vi "HFR500 Check comms.vi"(3 "Channel Name String":string) -> (1 "Comms Channel Number":i32)   [LabVIEW 2022 SP3]
uses:
  HFR500 ppm Range.ctl
  Globals/Meas_global.vi
panel:
  out "Testing Ch Number":i32
  out "Number of Black Box file reads":i32
  out "Channel  number with good response":i32[](array[numeric])
  out "Channel numbers being polled":i32
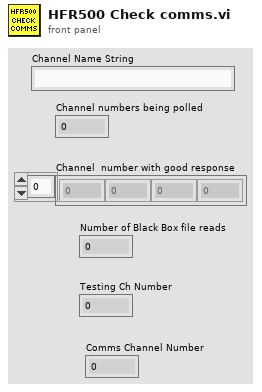
[diagram p1: front panel]
types:
  T1 = typedef "HFR500 ppm Range.ctl" = enum16{"None", "1,000", "2,000", "5,000", "10,000", "20,000", "50,000", "100,000", "200,000"}
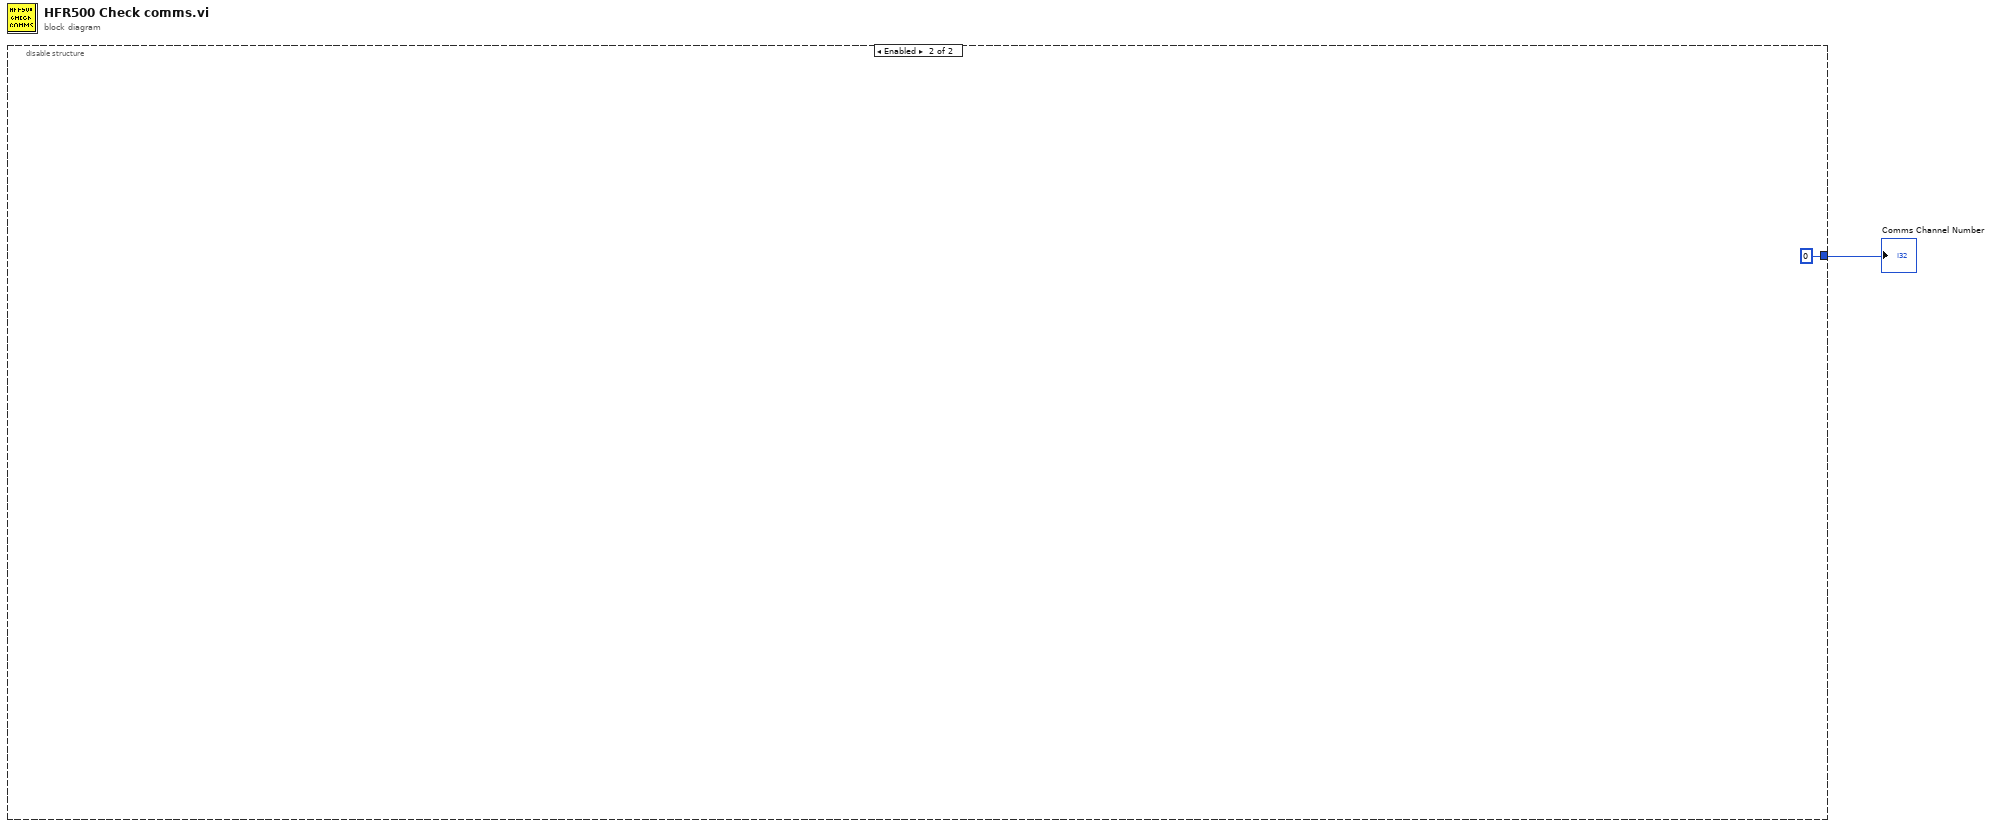
[diagram p0: block diagram]
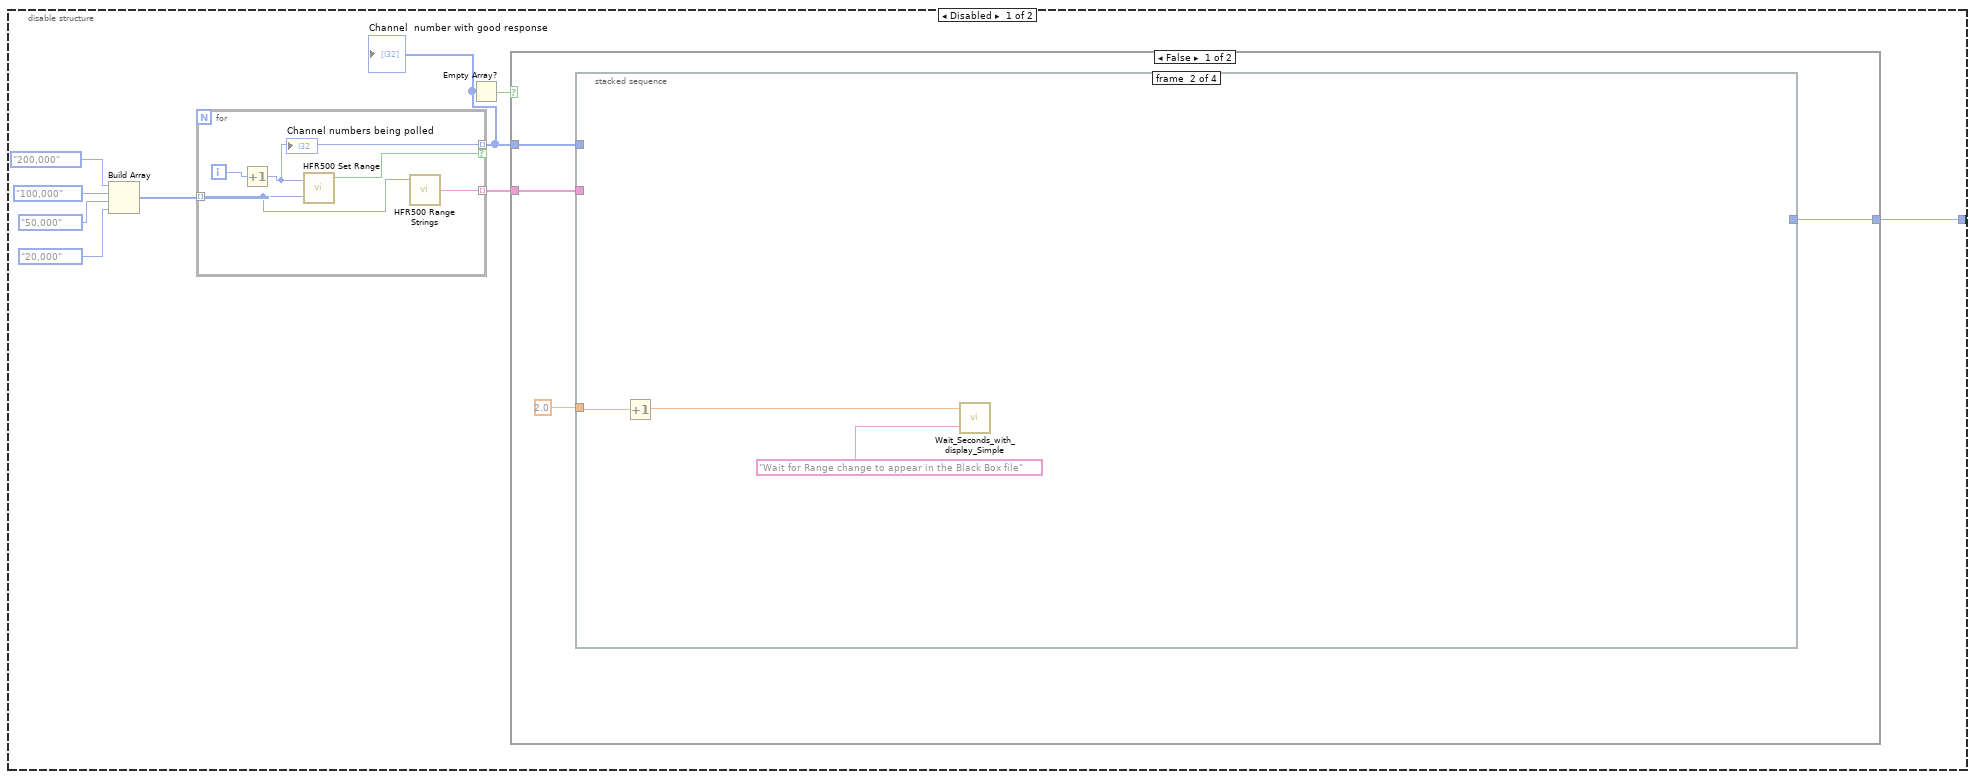
[diagram p2: hidden frame]
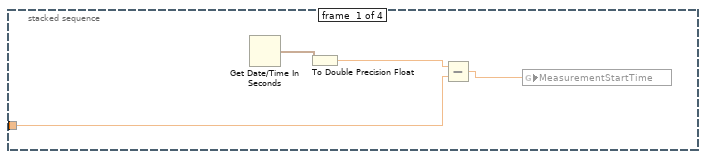
[diagram p3: hidden frame]
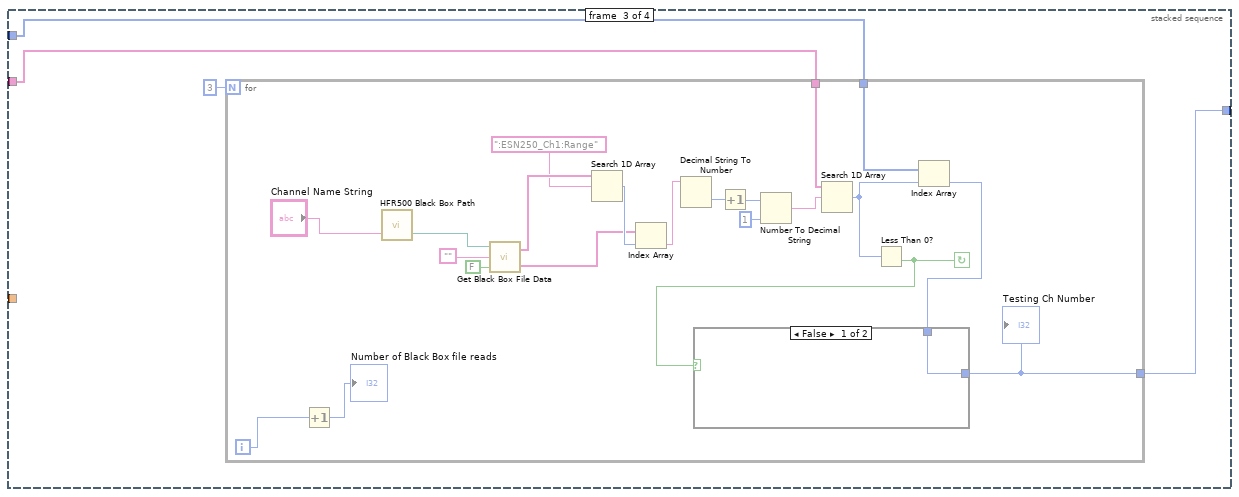
[diagram p4: hidden frame]
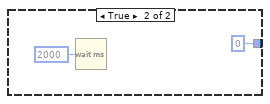
[diagram p5: hidden frame]
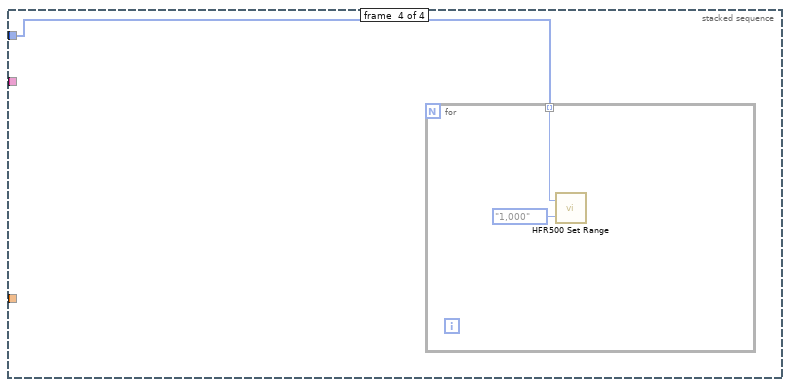
[diagram p6: hidden frame]
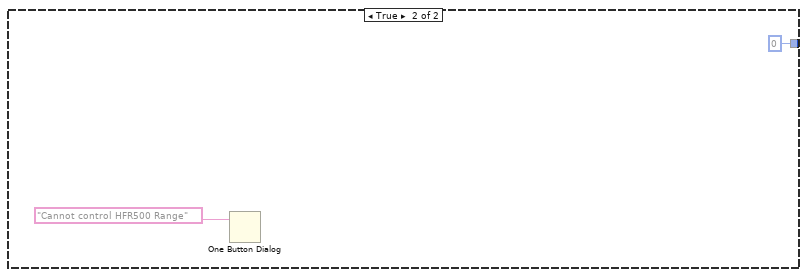
[diagram p7: hidden frame]
diagram:
  n1 = disable-structure shown="Enabled" {
    disable-tunnel: [w2 0 ("Comms Channel Number")] -> w1
    frame Disabled {
      n2 = Build Array(HFR500_ppm_Range."200,000" ("ppm Range"), HFR500_ppm_Range."100,000" ("ppm Range"), HFR500_ppm_Range."50,000" ("ppm Range"), HFR500_ppm_Range."20,000" ("ppm Range")) -> (w10:T1[])
      n3 = for {
        tunnel: w10 -> [w58] mode=indexing
        tunnel: [w57] -> w3 mode=indexing if=w56
        tunnel: [w55] -> w5 mode=indexing
        i -> [w59]
        n4 = Increment(x=w59) -> (x+1=w57:i32)
        "Channel numbers being polled" <- w57
        n5 = call "HFR500 Set Range.vi"("Ch number"=w57, "ppm Range"=w58) -> ("Correctly Set?"=w56:bool)  [unwired: 2 out]
        n6 = call "HFR500 Range Strings.vi"("ppm Range"=w58) -> ("Range Digit"=w55:string)  [unwired: 3 in, 1 out]
      }
      "Channel  number with good response" <- w3
      n7 = Empty Array?(array=w3) -> (empty?=w4:bool)
      n8 = case shown="False" w4 {
        tunnel: w3 -> [w13 _]
        tunnel: w5 -> [w12 _]
        tunnel: [w11 0] -> w2
        frame False {
          n9 = stacked-sequence {
            tunnel: 2.0 ("y") -> [w15 w21 _ _]
            tunnel: w13 -> [_ _ w24 w50]
            tunnel: w12 -> [_ _ w23 _]
            tunnel: [_ _ w22 _] -> w11
            frame #0 {
              n10 = Get Date/Time In Seconds() -> (seconds since 1Jan1904=w18:timestamp)
              n11 = To Double Precision Float(number=w18) -> (double precision float=w16:dbl)
              n12 = Subtract(x=w16, y=w15) -> (x-y=w17:dbl)
              n13 = global write "Meas_global.vi" "MeasurementStartTime"(w17) -> ()
            }
            frame #1 {
              n14 = Increment(x=w21) -> (x+1=w19:dbl)
              n15 = call "Wait_Seconds_with_display_Simple.vi"("Message"="Wait for Range change to appear in the Black Box file", "Seconds to wait"=w19) -> ()  [unwired: 1 in, 1 out]
            }
            frame #2 {
              n16 = for {
                N: 3 -> [_]
                tunnel: w23 -> [w38]
                tunnel: w24 -> [w37]
                tunnel: [w34] -> w22
                i -> [w27]
                stop <- w35 continue-if-true
                n17 = Increment(x=w27) -> (x+1=→"Number of Black Box file reads":i32)
                n18 = call "HFR500 Black Box Path.vi"("Channel Name String"="Channel Name String") -> ("Black Box Path"=w46:path)  [unwired: 1 in, 1 out]
                n19 = call "Get Black Box File Data.vi"("Delete File?"=FALSE, "Inst Name"="", "Black Box Filename"=w46) -> ("Channel Values"=w39:string[], "Channel Names"=w44:string[])
                n20 = Search 1D Array(1D array=w44, element=":ESN250_Ch1:Range") -> (index of element=w40:i32)  [unwired: 1 out]
                n21 = Index Array(array=w39, index=w40) -> (element=w32:string)
                n22 = Decimal String To Number(string=w32) -> (number=w31:i32)  [unwired: 2 in, 1 out]
                n23 = Increment(x=w31) -> (x+1=w30:i32)
                n24 = Number To Decimal String(number=w30, width (-)=i16 1) -> (decimal integer string=w29:string)
                n25 = Search 1D Array(1D array=w38, element=w29) -> (index of element=w36:i32)  [unwired: 1 out]
                n26 = Less Than 0?(x=w36) -> (x < 0?=w35:bool)
                n27 = Index Array(array=w37, index=w36) -> (element=w33:i32)
                n28 = case shown="False" w35 {
                  tunnel: [w47 0] -> w34
                  tunnel: w33 -> [w47 _]
                  frame False {
                  }
                  frame True {
                    n29 = Wait (ms)(milliseconds to wait=u32 2000) -> ()  [unwired: 1 out]
                  }
                }
                "Testing Ch Number" <- w34
              }
            }
            frame #3 {
              n30 = for {
                tunnel: w50 -> [w52] mode=indexing
                n31 = call "HFR500 Set Range.vi"("Ch number"=w52, "ppm Range"=HFR500_ppm_Range."1,000") -> ()  [unwired: 3 out]
              }
            }
          }
        }
        frame True {
          n32 = One Button Dialog(message="Cannot control HFR500 Range") -> ()  [unwired: 1 in, 1 out]
        }
      }
    }
    frame Enabled {
    }
  }
  "Comms Channel Number" <- w1
